vi "Reserve Hardware for Measurement.vi"(8 "error in (no error)":errorcluster, 10 "Hardware to Reserve":string, 11 "Controller in":refnum<class "Controller.lvclass">) -> (0 "error out":errorcluster, 3 "Controller out":refnum<class "Controller.lvclass">)   [LabVIEW 2016, in "Controller Actor.lvlib" / "Controller.lvclass"]
uses:
  Controller.lvclass
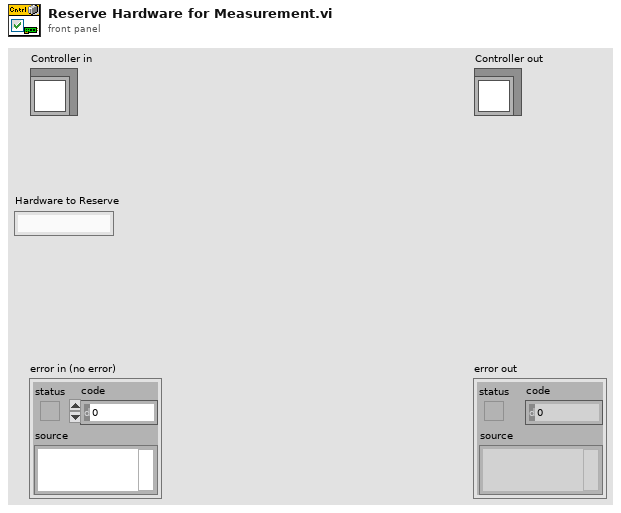
[diagram p1: front panel]
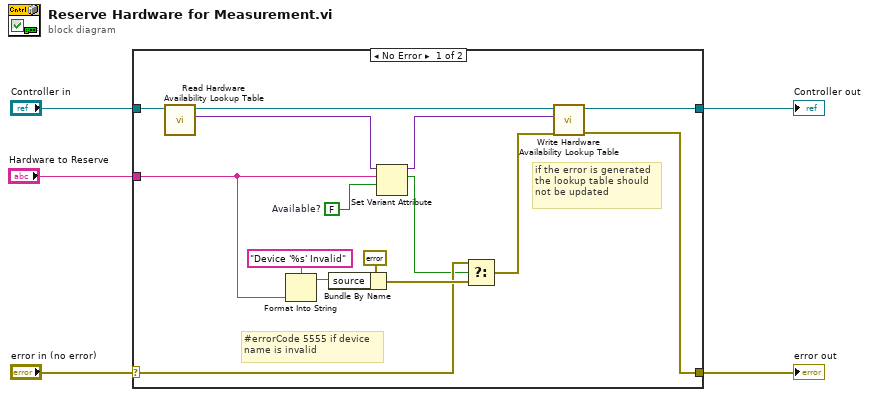
[diagram p0: block diagram]
diagram:
  n1 = case shown="No Error" "error in (no error)" {
    selector: "error in (no error)" -> [w9 w22]
    tunnel: [w6 w22] -> w4
    tunnel: [w15 w21] -> w2
    tunnel: "Controller in" -> [w18 w21]
    tunnel: "Hardware to Reserve" -> [w10 _]
    frame No Error {
      w19 = FALSE  # Available?
      # "if the error is generated\nthe lookup table should\nnot be updated"
      # "#errorCode 5555 if device\nname is invalid"
      n2 = call "Read Hardware Availability Lookup Table.vi"("Controller in"=w18) -> ("Hardware Availability Lookup Table"=w20:variant, "Controller out"=w17:refnum<class "Controller.lvclass">)  [unwired: 8 in, 1 out]
      n3 = Format Into String(format string="Device '%s' Invalid" ("source"), w10) -> (resulting string=w13:string)  [unwired: 2 in, 1 out]
      n4 = Bundle By Name(cluster=errorcluster {"status"=TRUE, "code"=5555, "source"="Device '%s' Invalid"} ("error constant"), "source"=w13) -> (w11:errorcluster)
      n5 = Set Variant Attribute(Variant=w20, name=w10, value=w19) -> (Variant out=w16:variant, replaced=w8:bool)  [unwired: 1 in, 1 out]
      n6 = Select(t=w9, s=w8, f=w11) -> (s? t:f=w7:errorcluster)
      n7 = call "Write Hardware Availability Lookup Table.vi"("error in (no error)"=w7, "Hardware Availability Lookup Table"=w16, "Controller in"=w17) -> ("error out"=w6:errorcluster, "Controller out"=w15:refnum<class "Controller.lvclass">)  [unwired: 7 in]
    }
    frame Error {
    }
  }
  "error out" <- w4
  "Controller out" <- w2
